vi "SID_adsr.vi"(0 "status in":T2(ring), 1 "Reg":T1 {"Duty" format="%0.2f"; "ADSR"."R" format="%0.2f"; "ADSR"."S" format="%0.2f"; "ADSR"."D" format="%0.2f"; "ADSR"."A" format="%0.2f"; "freq" format="%0.2f"}, 5 "mod in":dbl, 7 "acc in":dbl) -> (4 "status out":T2(ring), 6 "mod out":dbl, 8 "acc out":dbl)   [LabVIEW 2018]
uses:
  SID_voice_reg.ctl
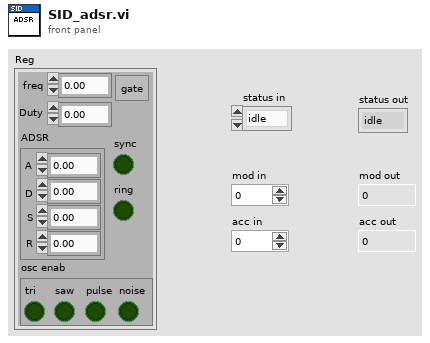
[diagram p1: front panel]
types:
  T1 = typedef "SID_voice_reg.ctl" = cluster{"freq":dbl, "gate":bool, "ADSR":cluster{"A":dbl, "D":dbl, "S":dbl, "R":dbl}, "Duty":dbl, "osc enab":cluster{"tri":bool, "saw":bool, "pulse":bool, "noise":bool}, "sync":bool, "ring":bool}
  T2 = enum16{"idle", "pre-attack", "attack", "pre-decay", "decay", "sustain", "pre-release", "release"}
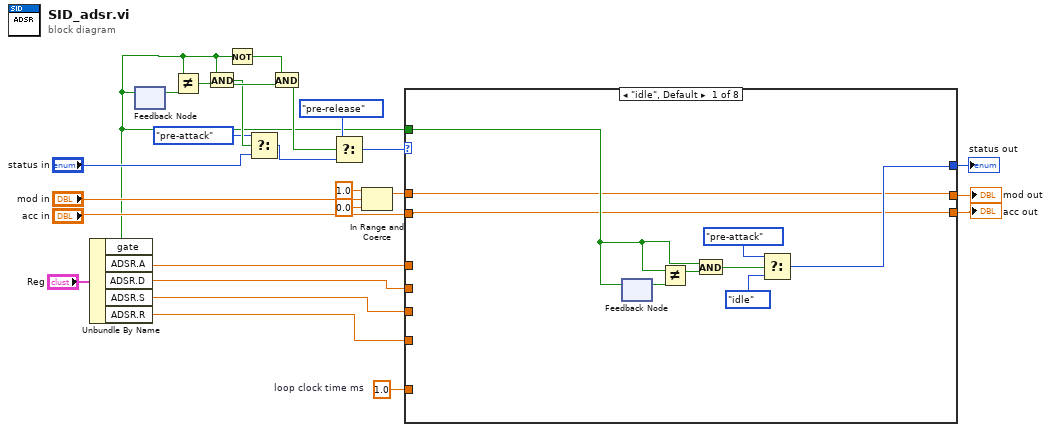
[diagram p0: block diagram]
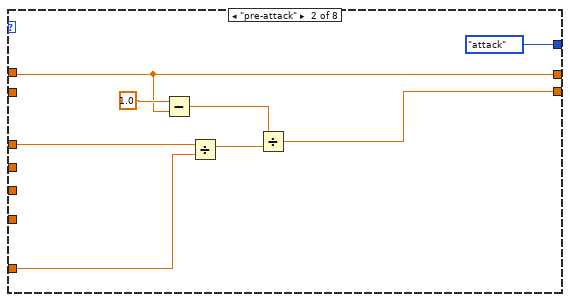
[diagram p2: hidden frame]
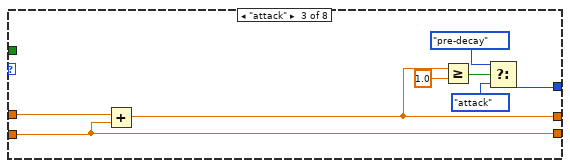
[diagram p3: hidden frame]
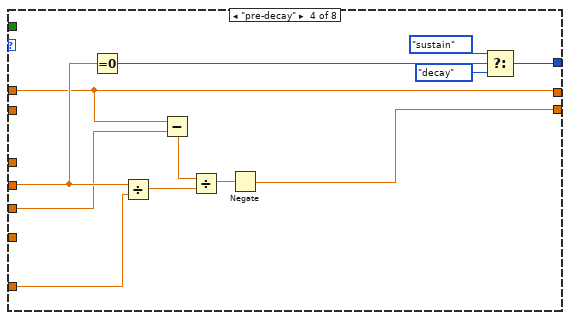
[diagram p4: hidden frame]
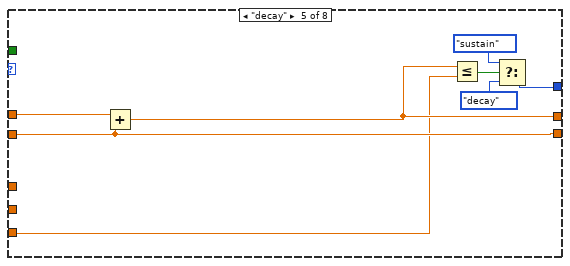
[diagram p5: hidden frame]
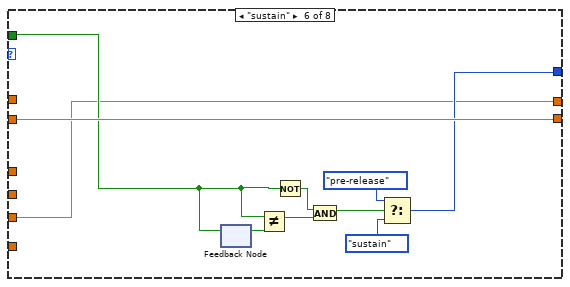
[diagram p6: hidden frame]
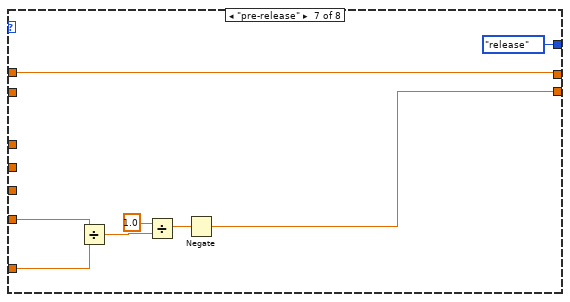
[diagram p7: hidden frame]
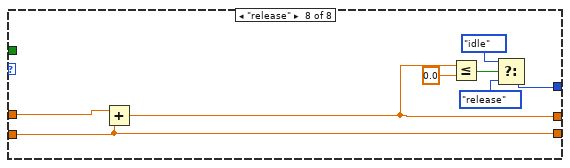
[diagram p8: hidden frame]
diagram:
  w11 = 1.0  # loop clock time ms
  n1 = Unbundle By Name("Reg") -> ("gate"=w1:bool, "ADSR.A"=w5:dbl, "ADSR.D"=w4:dbl, "ADSR.S"=w3:dbl, "ADSR.R"=w2:dbl)
  n2 = feedback #1() -> (w24:bool)  [unwired: 1 in]
  n3 = feedback-in #1(w1) -> ()
  n4 = Not Equal?(x=w1, y=w24) -> (x != y?=w23:bool)
  n5 = And(x=w1, y=w23) -> (x .and. y?=w21:bool)
  n6 = Not(x=w1) -> (.not. x?=w22:bool)
  n7 = Select(t=T2."pre-attack", s=w21, f="status in") -> (s? t:f=w17:T2)
  n8 = And(x=w22, y=w23) -> (x .and. y?=w12:bool)
  n9 = Select(t=T2."pre-release", s=w12, f=w17) -> (s? t:f=w20:T2)
  n10 = In Range and Coerce(upper limit=1.0, x="mod in", lower limit=0.0) -> (coerced(x)=w13:dbl)  [unwired: 1 out]
  n11 = case shown="\"idle\", Default" w20 {
    tunnel: [w26 w42 w49 w60 w69 w80 w82 w90] -> w7
    tunnel: "acc in" -> [w26 _ w49 _ w69 w80 _ w90]
    tunnel: w13 -> [w27 w36 w50 w53 w70 _ w87 w92]
    tunnel: [w27 w36 w48 w53 w65 w71 w87 w89] -> w9
    tunnel: [w29 T2."attack" w43 w57 w63 w72 T2."release" w91] -> w25
    tunnel: w1 -> [w28 _ _ _ _ w77 _ _]
    tunnel: w5 -> [_ w39 _ _ _ _ _ _]
    tunnel: w4 -> [_ _ _ w59 _ _ _ _]
    tunnel: w3 -> [_ _ _ w52 w64 w71 _ _]
    tunnel: w2 -> [_ _ _ _ _ _ w83 _]
    tunnel: w11 -> [_ w38 _ w54 _ _ w81 _]
    frame "idle", Default {
      n12 = feedback #2() -> (w34:bool)  [unwired: 1 in]
      n13 = feedback-in #2(w28) -> ()
      n14 = Not Equal?(x=w28, y=w34) -> (x != y?=w33:bool)
      n15 = And(x=w28, y=w33) -> (x .and. y?=w32:bool)
      n16 = Select(t=T2."pre-attack", s=w32, f=T2."idle") -> (s? t:f=w29:T2)
    }
    frame "pre-attack" {
      n17 = Subtract(x=1.0 ("y"), y=w36) -> (x-y=w35:dbl)
      n18 = Divide(x=w39, y=w38) -> (x/y=w41:dbl)
      n19 = Divide(x=w35, y=w41) -> (x/y=w42:dbl)
    }
    frame "attack" {
      n20 = Add(x=w50, y=w49) -> (x+y=w48:dbl)
      n21 = Greater Or Equal?(x=w48, y=1.0) -> (x >= y?=w44:bool)
      n22 = Select(t=T2."pre-decay", s=w44, f=T2."attack") -> (s? t:f=w43:T2)
    }
    frame "pre-decay" {
      n23 = Equal To 0?(x=w59) -> (x = 0?=w56:bool)
      n24 = Divide(x=w59, y=w54) -> (x/y=w62:dbl)
      n25 = Subtract(x=w53, y=w52) -> (x-y=w51:dbl)
      n26 = Divide(x=w51, y=w62) -> (x/y=w61:dbl)
      n27 = Negate(x=w61) -> (-x=w60:dbl)
      n28 = Select(t=T2."sustain", s=w56, f=T2."decay") -> (s? t:f=w57:T2)
    }
    frame "decay" {
      n29 = Add(x=w70, y=w69) -> (x+y=w65:dbl)
      n30 = Less Or Equal?(x=w65, y=w64) -> (x <= y?=w66:bool)
      n31 = Select(t=T2."sustain", s=w66, f=T2."decay") -> (s? t:f=w63:T2)
    }
    frame "sustain" {
      n32 = feedback #3() -> (w79:bool)  [unwired: 1 in]
      n33 = feedback-in #3(w77) -> ()
      n34 = Not Equal?(x=w77, y=w79) -> (x != y?=w78:bool)
      n35 = Not(x=w77) -> (.not. x?=w76:bool)
      n36 = And(x=w76, y=w78) -> (x .and. y?=w73:bool)
      n37 = Select(t=T2."pre-release", s=w73, f=T2."sustain") -> (s? t:f=w72:T2)
    }
    frame "pre-release" {
      n38 = Divide(x=w83, y=w81) -> (x/y=w85:dbl)
      n39 = Divide(x=1.0 ("y"), y=w85) -> (x/y=w84:dbl)
      n40 = Negate(x=w84) -> (-x=w82:dbl)
    }
    frame "release" {
      n41 = Add(x=w92, y=w90) -> (x+y=w89:dbl)
      n42 = Less Or Equal?(x=w89, y=0.0) -> (x <= y?=w95:bool)
      n43 = Select(t=T2."idle", s=w95, f=T2."release") -> (s? t:f=w91:T2)
    }
  }
  "status out" <- w25
  "mod out" <- w9
  "acc out" <- w7
